vi "TCP Client_34.vi"(0 "CMD":i32(ring) items=["OCP_IF_CMD_TRACE_READ", "OCP_IF_CMD_TRACE_RESET", "OCP_IF_CMD_TRACE_GET_SIZE", "OCP_IF_CMD_TRACE_SET_SIZE", "OCP_IF_CMD_TRACE_GET_NUMBER_SIGNALS", "OCP_IF_CMD_TRACE_GET_SIGNALS_NAMES", "OCP_IF_CMD_TRACE_GET_NUMBER_TRACES", "OCP_IF_CMD_TRACE_GET_TRACES_NAMES", "OCP_IF_CMD_TRACE_GET_ADDRESS", "OCP_IF_CMD_CS_STATUS", "OCP_IF_CMD_CS_ENABLE", "OCP_IF_CMD_CS_DISABLE", "OCP_IF_CMD_CS_CONTROLLER_IF", "OCP_IF_CMD_CS_HARDWARE_IF", "OCP_IF_CMD_CS_GET_NUMBER_CONTROLLERS", "OCP_IF_CMD_CS_GET_CONTROLLERS_NAMES", "OCP_IF_CMD_PLATFORM_ID", "OCP_IF_CMD_PLATFORM_IF", "OCP_IF_CMD_OPIL_UPDATE_MEASUREMENTS", "OCP_IF_CMD_OPIL_UPDATE_SIM_DATA", "OCP_IF_CMD_OPIL_RUN_CONTROL", "OCP_IF_CMD_OPIL_INITIALIZE_CONTROL", "OCP_IF_CMD_OPIL_GET_CONTROL", "OCP_IF_CMD_OPIL_GET_CONTROLLER_DATA", "OCP_IF_CMD_END"], 2 "Input Cluster":T3, 3 "error in (no error)":errorcluster, 8 "Comunication Cluster":T1) -> (6 "Output cluster":T2, 7 "R_message 1":string, 10 "error out":errorcluster)   [LabVIEW 2021]
uses:
  <vilib>/ErrorRing/Error Ring.xnode
  <vilib>/Utility/error.llb/Error Cluster From Error Code.vi
panel:
  out "R_Data string length":cluster{i32}
  out "W_Data string length: \nbytes written 2":i32
  out "W_Data string_flat":string
  # "0-> OCP_IF_CMD_TRACE_READ = 0, //LV: SIZE - CMD - ID || RESPONSE: SIZE - DATA\n1->\tOCP_IF_CMD_TRACE_RESET, //SIZE - CMD - ID || RESPONSE: SIZE\n2-> OCP_IF_CMD_TRACE_GET_SIZE, //SIZE - CMD - ID || RESPONSE: SIZE - TRACE_SIZE (4 bztes)\n3->\tOCP_IF_CMD_TRACE_SET_SIZE, //SIZE - CMD - ID - TRACE_SIZE ( 4 bytes) || RESPONSE: SIZE\n4->\tOCP_IF_CMD_TRACE_GET_NUMBER_SIGNALS, //SIZE - CMD - ID || RESPONSE: SIZE - NB_SIGNALS (4 bytes)\n5->\tOCP_IF_CMD_TRACE_GET_SIGNALS_NAMES, //SIZE - CMD - ID || RESPONSE: SIZE - string\n6->\tOCP_IF_CMD_TRACE_GET_NUMBER_TRACES, //SIZE - CMD  || RESPONSE: SIZE - NB_TRACES (4 bytes)\n7->\tOCP_IF_CMD_TRACE_GET_TRACES_NAMES, //SIZE - CMD || RESPONSE: SIZE - NB_TRACES (N bytes)\n8-> OCP_IF_CMD_TRACE_GET_ADDRESS, //SIZE - CMD - ID || RESPONSE: SIZE - TRACE ADDRESS (4 bytes)\n9-> OCP_IF_CMD_CS_STATUS, //SIZE - CMD - ID || RESPONSE: SIZE - CS STATUS (4 bytes)\n10-> OCP_IF_CMD_CS_ENABLE, //SIZE - CMD - ID || RESPONSE: SIZE\n11-> OCP_IF_CMD_CS_DISABLE, //SIZE - CMD - ID || RESPONSE: SIZE\n12-> OCP_IF_CMD_CS_CONTROLLER_IF, //SIZE - CMD - ID - DATA (N) || RESPONSE: SIZE - DATA (M)\n13-> OCP_IF_CMD_CS_HARDWARE_IF, //SIZE - CMD - ID - DATA (N) || RESPONSE: SIZE - DATA (M)\n14-> OCP_IF_CMD_CS_GET_NUMBER_CONTROLLERS, //SIZE - CMD || RESPONSE: SIZE - NB CSs\n15-> OCP_IF_CMD_CS_GET_CONTROLLERS_NAMES, //SIZE - CMD || RESPONSE: SIZE - string NAMES CSs"
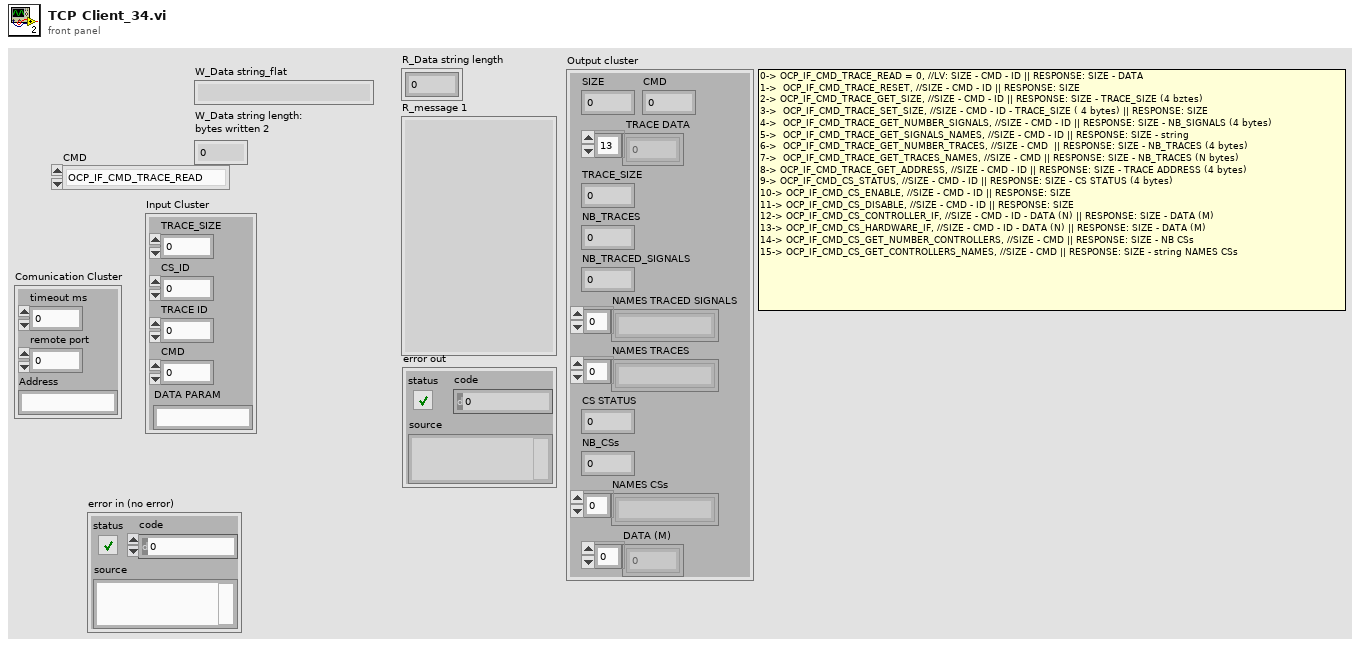
[diagram p1: front panel]
types:
  T1 = cluster{"timeout ms":i32, "remote port":u16, "Address":string}
  T2 = cluster{"SIZE":i32, " TRACE DATA":sgl[], "TRACE_SIZE":i32, "NB_TRACES":i32, "NB_TRACED_SIGNALS":i32, "NAMES TRACED SIGNALS":string[], "NAMES TRACES":string[], "CS STATUS":i32, "NB_CSs":i32, "NAMES CSs":string[], "DATA (M)":sgl[], "CMD":i32}
  T3 = cluster{"TRACE_SIZE":i32, "CS_ID":i32, "TRACE ID":i32, "CMD":i32, "DATA PARAM":string}
  T4 = enum16{"big-endian, network order", "native, host order", "little-endian"}
  T5 = enum16{"Standard", "Buffered", "CRLF", "Immediate"}
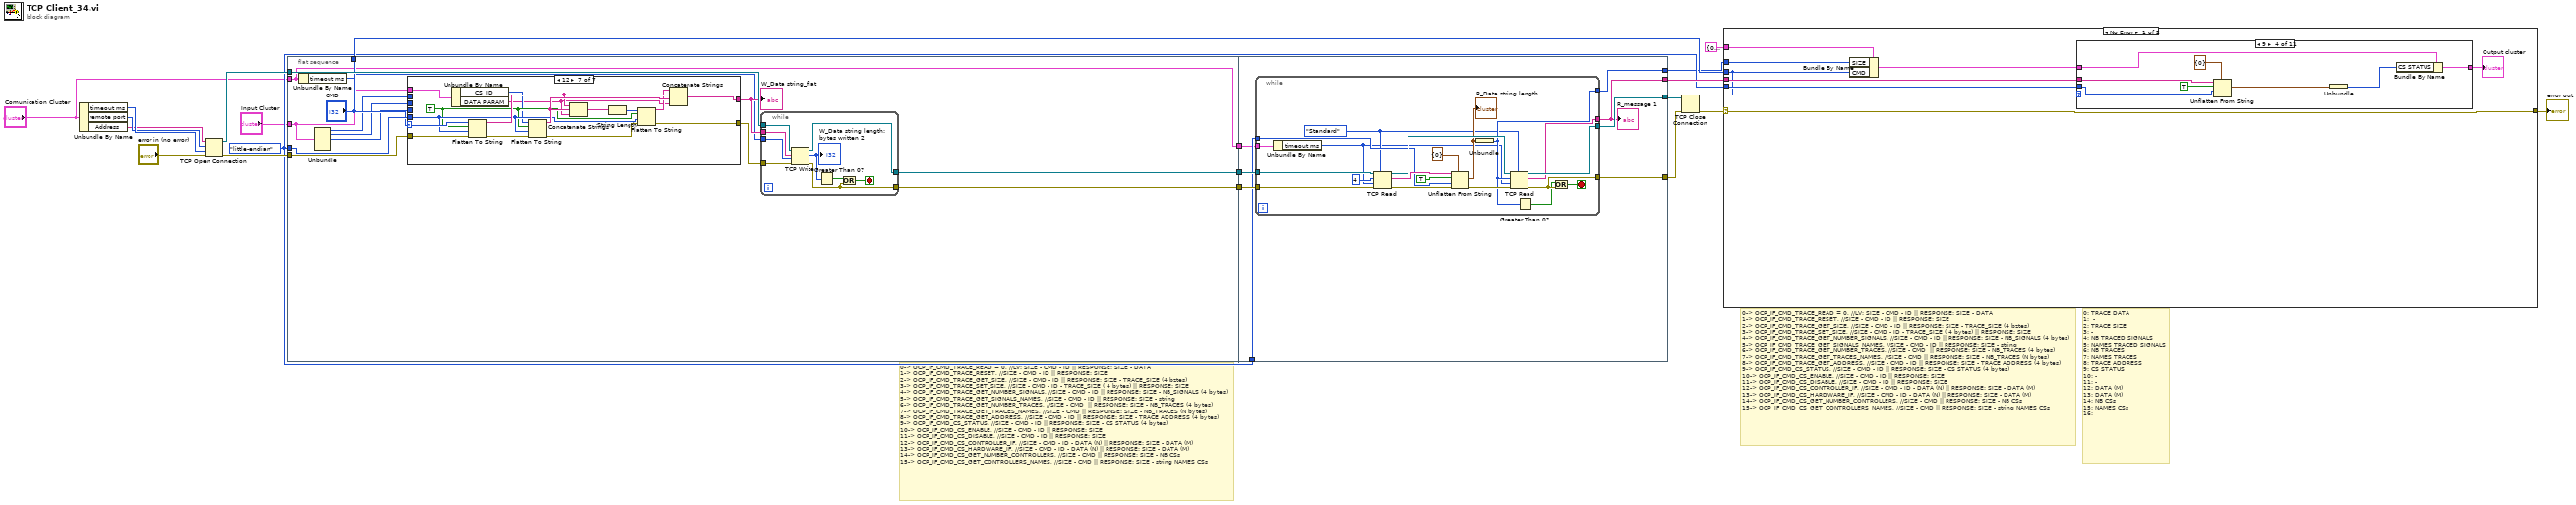
[diagram p0: block diagram]
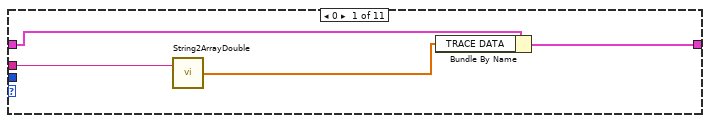
[diagram p2: hidden frame]
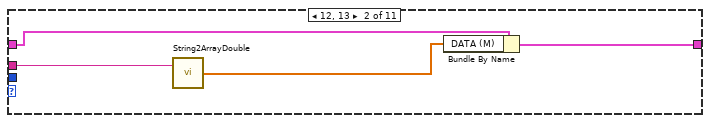
[diagram p3: hidden frame]
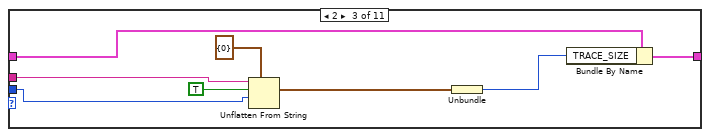
[diagram p4: hidden frame]
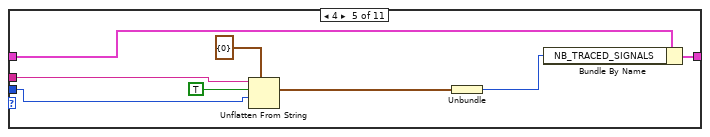
[diagram p5: hidden frame]
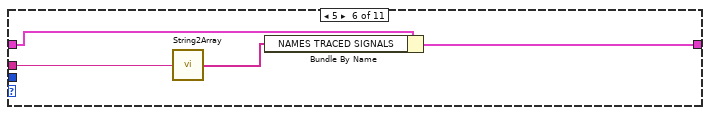
[diagram p6: hidden frame]
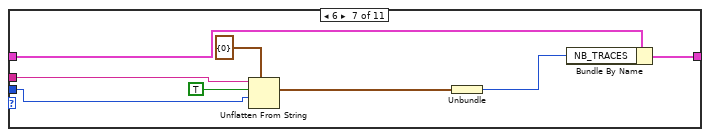
[diagram p7: hidden frame]
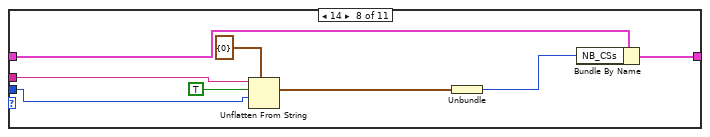
[diagram p8: hidden frame]
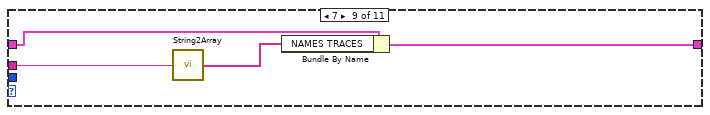
[diagram p9: hidden frame]
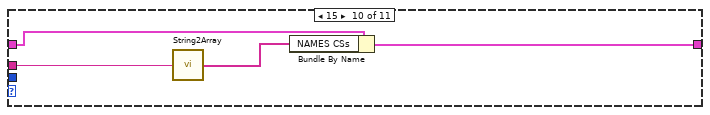
[diagram p10: hidden frame]
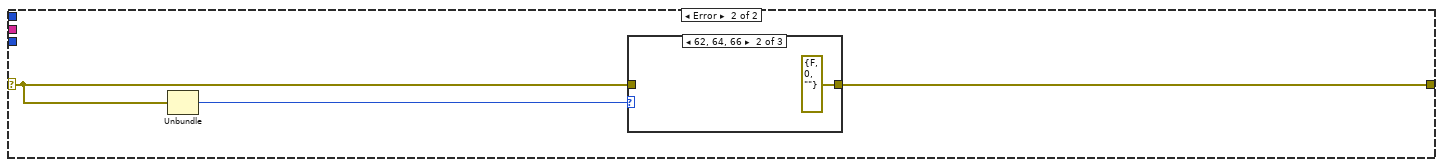
[diagram p12: hidden frame]
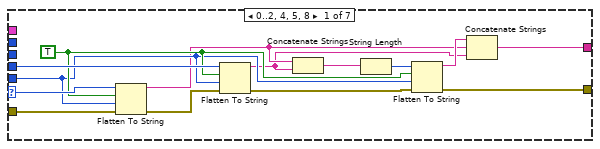
[diagram p15: hidden frame]
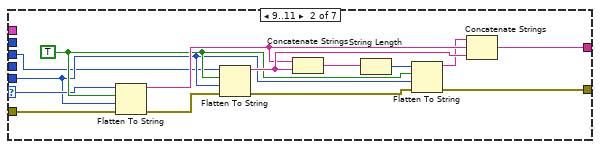
[diagram p16: hidden frame]
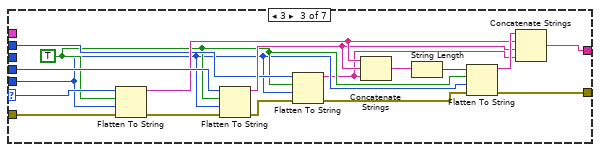
[diagram p17: hidden frame]
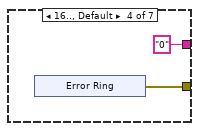
[diagram p18: hidden frame]
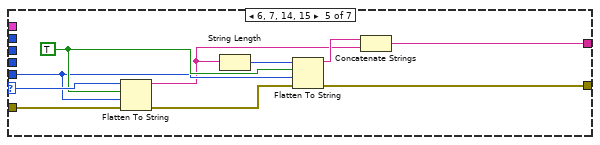
[diagram p19: hidden frame]
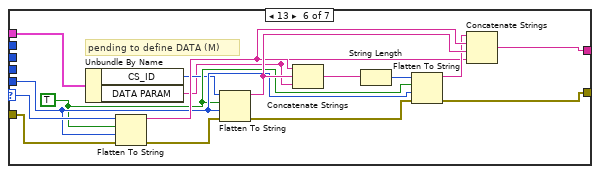
[diagram p20: hidden frame]
diagram:
  w8 = T4."little-endian" ("byte order (0:big-endian, network order)")
  # "0-> OCP_IF_CMD_TRACE_READ = 0, //LV: SIZE - CMD - ID || RESPONSE: SIZE - DATA\n1->\tOCP_IF_CMD_TRACE_RESET, //SIZE - CMD - ID || RESPONSE: SIZE\n2-> OCP_IF_CMD_TRACE_GET_SIZE, //SIZE - CMD - ID || RESPONSE: SIZE - TRACE_SIZE (4 bztes)\n3->\tOCP_IF_CMD_TRACE_SET_SIZE, //SIZE - CMD - ID - TRACE_SIZE ( 4 bytes) || RESPONSE: SIZE\n4->\tOCP_IF_CMD_TRACE_GET_NUMBER_SIGNALS, //SIZE - CMD - ID || RESPONSE: SIZE - NB_SIGNALS (4 bytes)\n5->\tOCP_IF_CMD_TRACE_GET_SIGNALS_NAMES, //SIZE - CMD - ID || RESPONSE: SIZE - string\n6->\tOCP_IF_CMD_TRACE_GET_NUMBER_TRACES, //SIZE - CMD  || RESPONSE: SIZE - NB_TRACES (4 bytes)\n7->\tOCP_IF_CMD_TRACE_GET_TRACES_NAMES, //SIZE - CMD || RESPONSE: SIZE - NB_TRACES (N bytes)\n8-> OCP_IF_CMD_TRACE_GET_ADDRESS, //SIZE - CMD - ID || RESPONSE: SIZE - TRACE ADDRESS (4 bytes)\n9-> OCP_IF_CMD_CS_STATUS, //SIZE - CMD - ID || RESPONSE: SIZE - CS STATUS (4 bytes)\n10-> OCP_IF_CMD_CS_ENABLE, //SIZE - CMD - ID || RESPONSE: SIZE\n11-> OCP_IF_CMD_CS_DISABLE, //SIZE - CMD - ID || RESPONSE: SIZE\n12-> OCP_IF_CMD_CS_CONTROLLER_IF, //SIZE - CMD - ID - DATA (N) || RESPONSE: SIZE - DATA (M)\n13-> OCP_IF_CMD_CS_HARDWARE_IF, //SIZE - CMD - ID - DATA (N) || RESPONSE: SIZE - DATA (M)\n14-> OCP_IF_CMD_CS_GET_NUMBER_CONTROLLERS, //SIZE - CMD || RESPONSE: SIZE - NB CSs\n15-> OCP_IF_CMD_CS_GET_CONTROLLERS_NAMES, //SIZE - CMD || RESPONSE: SIZE - string NAMES CSs"
  # "0: TRACE DATA\n1:  -\n2: TRACE SIZE\n3: -\n4: NB TRACED SIGNALS\n5: NAMES TRACED SIGNALS\n6: NB TRACES\n7: NAMES TRACES\n8: TRACE ADDRESS\n9: CS STATUS\n10: -\n11: -\n12: DATA (M)\n13: DATA (M)\n14: NB CSs \n15: NAMES CSs \n16:"
  # "0-> OCP_IF_CMD_TRACE_READ = 0, //LV: SIZE - CMD - ID || RESPONSE: SIZE - DATA\n1->\tOCP_IF_CMD_TRACE_RESET, //SIZE - CMD - ID || RESPONSE: SIZE\n2-> OCP_IF_CMD_TRACE_GET_SIZE, //SIZE - CMD - ID || RESPONSE: SIZE - TRACE_SIZE (4 bztes)\n3->\tOCP_IF_CMD_TRACE_SET_SIZE, //SIZE - CMD - ID - TRACE_SIZE ( 4 bytes) || RESPONSE: SIZE\n4->\tOCP_IF_CMD_TRACE_GET_NUMBER_SIGNALS, //SIZE - CMD - ID || RESPONSE: SIZE - NB_SIGNALS (4 bytes)\n5->\tOCP_IF_CMD_TRACE_GET_SIGNALS_NAMES, //SIZE - CMD - ID || RESPONSE: SIZE - string\n6->\tOCP_IF_CMD_TRACE_GET_NUMBER_TRACES, //SIZE - CMD  || RESPONSE: SIZE - NB_TRACES (4 bytes)\n7->\tOCP_IF_CMD_TRACE_GET_TRACES_NAMES, //SIZE - CMD || RESPONSE: SIZE - NB_TRACES (N bytes)\n8-> OCP_IF_CMD_TRACE_GET_ADDRESS, //SIZE - CMD - ID || RESPONSE: SIZE - TRACE ADDRESS (4 bytes)\n9-> OCP_IF_CMD_CS_STATUS, //SIZE - CMD - ID || RESPONSE: SIZE - CS STATUS (4 bytes)\n10-> OCP_IF_CMD_CS_ENABLE, //SIZE - CMD - ID || RESPONSE: SIZE\n11-> OCP_IF_CMD_CS_DISABLE, //SIZE - CMD - ID || RESPONSE: SIZE\n12-> OCP_IF_CMD_CS_CONTROLLER_IF, //SIZE - CMD - ID - DATA (N) || RESPONSE: SIZE - DATA (M)\n13-> OCP_IF_CMD_CS_HARDWARE_IF, //SIZE - CMD - ID - DATA (N) || RESPONSE: SIZE - DATA (M)\n14-> OCP_IF_CMD_CS_GET_NUMBER_CONTROLLERS, //SIZE - CMD || RESPONSE: SIZE - NB CSs\n15-> OCP_IF_CMD_CS_GET_CONTROLLERS_NAMES, //SIZE - CMD || RESPONSE: SIZE - string NAMES CSs"
  n1 = Unbundle By Name("Comunication Cluster") -> ("timeout ms"=w4:i32, "remote port"=w3:u16, "Address"=w2:string)
  n2 = TCP Open Connection(address=w2, remote port or service name=w3, timeout ms (60000)=w4, error in (no error)="error in (no error)") -> (connection ID=w20:refnum<k5>, error out=w19:errorcluster)  [unwired: 1 in]
  n3 = flat-sequence {
    tunnel: w20 -> [w34]
    tunnel: w19 -> [w31]
    tunnel: [w33] -> w18
    tunnel: [w32] -> w17
    tunnel: w8 -> [w30]
    tunnel: ["CMD"] -> w11
    tunnel: "Input Cluster" -> [w24]
    tunnel: "Comunication Cluster" -> [w22]
    tunnel: [w22] -> w1
    tunnel: w18 -> [w145]
    tunnel: w17 -> [w144]
    tunnel: [w143] -> w14
    tunnel: [w142] -> w13
    tunnel: w8 -> [w141]
    tunnel: [w140] -> w10
    tunnel: [w139] -> w7
    tunnel: w1 -> [w138]
    frame #0 {
      n4 = Unbundle By Name(w22) -> ("timeout ms"=w23:i32)
      n5 = Unbundle(w24) -> ("TRACE_SIZE"=w25:i32, "CS_ID"=w27:i32, "TRACE ID"=w26:i32)  [unwired: 2 out]
      n6 = case shown="12" "CMD" {
        selector: "CMD" -> [w55 w62 w86 _ w104 w113 w129]
        tunnel: w31 -> [w57 w63 w88 _ w105 w112 w128]
        tunnel: w30 -> [w48 w61 w74 _ w100 w109 w125]
        tunnel: w26 -> [w54 _ w85 _ _ _ _]
        tunnel: [w47 w59 w81 "0" w99 w115 w131] -> w29
        tunnel: [w46 w58 w73 w90 w97 w114 w130] -> w21
        tunnel: w25 -> [_ _ w76 _ _ _ _]
        tunnel: w27 -> [_ w60 _ _ _ _ _]
        tunnel: w24 -> [_ _ _ _ _ w111 w127]
        frame 0..2, 4, 5, 8 {
          w49 = TRUE ("prepend array or string size? (T)")
          n7 = Flatten To String(anything=w55, prepend array or string size? (T)=w49, byte order (0:big-endian, network order)=w48, error in (no error)=w57) -> (data string=w45:string, error out=w56:errorcluster)  [unwired: 1 out]
          n8 = Flatten To String(anything=w54, prepend array or string size? (T)=w49, byte order (0:big-endian, network order)=w48, error in (no error)=w56) -> (data string=w44:string, error out=w51:errorcluster)  [unwired: 1 out]
          n9 = Concatenate Strings(w45, w44) -> (w53:string)
          n10 = String Length(string=w53) -> (length=w52:i32)
          n11 = Flatten To String(anything=w52, prepend array or string size? (T)=w49, byte order (0:big-endian, network order)=w48, error in (no error)=w51) -> (data string=w50:string, error out=w46:errorcluster)  [unwired: 1 out]
          n12 = Concatenate Strings(w50, w45, w44) -> (w47:string)
        }
        frame 9..11 {
          w64 = TRUE ("prepend array or string size? (T)")
          n13 = Flatten To String(anything=w62, prepend array or string size? (T)=w64, byte order (0:big-endian, network order)=w61, error in (no error)=w63) -> (data string=w70:string, error out=w65:errorcluster)  [unwired: 1 out]
          n14 = Flatten To String(anything=w60, prepend array or string size? (T)=w64, byte order (0:big-endian, network order)=w61, error in (no error)=w65) -> (data string=w71:string, error out=w68:errorcluster)  [unwired: 1 out]
          n15 = Concatenate Strings(w70, w71) -> (w66:string)
          n16 = String Length(string=w66) -> (length=w67:i32)
          n17 = Flatten To String(anything=w67, prepend array or string size? (T)=w64, byte order (0:big-endian, network order)=w61, error in (no error)=w68) -> (data string=w69:string, error out=w58:errorcluster)  [unwired: 1 out]
          n18 = Concatenate Strings(w69, w70, w71) -> (w59:string)
        }
        frame 3 {
          w75 = TRUE ("prepend array or string size? (T)")
          n19 = Flatten To String(anything=w86, prepend array or string size? (T)=w75, byte order (0:big-endian, network order)=w74, error in (no error)=w88) -> (data string=w80:string, error out=w87:errorcluster)  [unwired: 1 out]
          n20 = Flatten To String(anything=w85, prepend array or string size? (T)=w75, byte order (0:big-endian, network order)=w74, error in (no error)=w87) -> (data string=w79:string, error out=w78:errorcluster)  [unwired: 1 out]
          n21 = Flatten To String(anything=w76, prepend array or string size? (T)=w75, byte order (0:big-endian, network order)=w74, error in (no error)=w78) -> (data string=w72:string, error out=w77:errorcluster)  [unwired: 1 out]
          n22 = Concatenate Strings(w80, w79, w72) -> (w84:string)
          n23 = String Length(string=w84) -> (length=w83:i32)
          n24 = Flatten To String(anything=w83, prepend array or string size? (T)=w75, byte order (0:big-endian, network order)=w74, error in (no error)=w77) -> (data string=w82:string, error out=w73:errorcluster)  [unwired: 1 out]
          n25 = Concatenate Strings(w82, w80, w79, w72) -> (w81:string)
        }
        frame 16.., Default {
          n26 = xnode "Error Ring"() -> ("error out"=w90:errorcluster)
        }
        frame 6, 7, 14, 15 {
          w101 = TRUE ("prepend array or string size? (T)")
          n27 = Flatten To String(anything=w104, prepend array or string size? (T)=w101, byte order (0:big-endian, network order)=w100, error in (no error)=w105) -> (data string=w96:string, error out=w98:errorcluster)  [unwired: 1 out]
          n28 = String Length(string=w96) -> (length=w103:i32)
          n29 = Flatten To String(anything=w103, prepend array or string size? (T)=w101, byte order (0:big-endian, network order)=w100, error in (no error)=w98) -> (data string=w102:string, error out=w97:errorcluster)  [unwired: 1 out]
          n30 = Concatenate Strings(w102, w96) -> (w99:string)
        }
        frame 13 {
          w108 = TRUE ("prepend array or string size? (T)")
          # "pending to define DATA (M)"
          n31 = Unbundle By Name(w111) -> ("CS_ID"=w107:i32, "DATA PARAM"=w106:string)
          n32 = Flatten To String(anything=w113, prepend array or string size? (T)=w108, byte order (0:big-endian, network order)=w109, error in (no error)=w112) -> (data string=w120:string, error out=w116:errorcluster)  [unwired: 1 out]
          n33 = Flatten To String(anything=w107, prepend array or string size? (T)=w108, byte order (0:big-endian, network order)=w109, error in (no error)=w116) -> (data string=w121:string, error out=w110:errorcluster)  [unwired: 1 out]
          n34 = Concatenate Strings(w120, w121, w106) -> (w117:string)
          n35 = String Length(string=w117) -> (length=w118:i32)
          n36 = Flatten To String(anything=w118, prepend array or string size? (T)=w108, byte order (0:big-endian, network order)=w109, error in (no error)=w110) -> (data string=w119:string, error out=w114:errorcluster)  [unwired: 1 out]
          n37 = Concatenate Strings(w119, w120, w121, w106) -> (w115:string)
        }
        frame 12 {
          w124 = TRUE ("prepend array or string size? (T)")
          n38 = Unbundle By Name(w127) -> ("CS_ID"=w123:i32, "DATA PARAM"=w122:string)
          n39 = Flatten To String(anything=w129, prepend array or string size? (T)=w124, byte order (0:big-endian, network order)=w125, error in (no error)=w128) -> (data string=w136:string, error out=w132:errorcluster)  [unwired: 1 out]
          n40 = Flatten To String(anything=w123, prepend array or string size? (T)=w124, byte order (0:big-endian, network order)=w125, error in (no error)=w132) -> (data string=w137:string, error out=w126:errorcluster)  [unwired: 1 out]
          n41 = Concatenate Strings(w136, w137, w122) -> (w133:string)
          n42 = String Length(string=w133) -> (length=w134:i32)
          n43 = Flatten To String(anything=w134, prepend array or string size? (T)=w124, byte order (0:big-endian, network order)=w125, error in (no error)=w126) -> (data string=w135:string, error out=w130:errorcluster)  [unwired: 1 out]
          n44 = Concatenate Strings(w135, w136, w137, w122) -> (w131:string)
        }
      }
      "W_Data string_flat" <- w29
      n45 = while {
        tunnel: w29 -> [w41]
        tunnel: w23 -> [w40]
        tunnel: w21 -> [w39]
        tunnel: [w37] -> w33
        tunnel: w34 -> [w43]
        tunnel: [w42] -> w32
        stop <- w38 stop-if-true
        n46 = TCP Write(connection ID=w43, data in=w41, error in (no error)=w39, 9:w40) -> (connection ID out=w42:refnum<k5>, bytes written=w36:i32, error out=w37:errorcluster)
        "W_Data string length: \nbytes written 2" <- w36
        n47 = Greater Than 0?(x=w36) -> (x > 0?=w35:bool)
        n48 = Or(x=w35, y=w37) -> (x .or. y?=w38:bool)
      }
    }
    frame #1 {
      n49 = while {
        tunnel: w141 -> [w155]
        tunnel: [w153] -> w140
        tunnel: [w150] -> w139
        tunnel: w144 -> [w163]
        tunnel: [w162] -> w143
        tunnel: w145 -> [w164]
        tunnel: [w152] -> w142
        tunnel: w138 -> [w146]
        stop <- w151 stop-if-true
        w148 = T5."Standard" ("mode (standard)")
        n50 = Unbundle By Name(w146) -> ("timeout ms"=w147:i32)
        n51 = TCP Read(connection ID=w163, bytes to read=4, error in (no error)=w164, 7:w148, 9:w147) -> (connection ID out=w165:refnum<k5>, data out=w161:string, error out=w157:errorcluster)
        n52 = Unflatten From String(type=cluster{i32} {0}, binary string=w161, data includes array or string size? (T)=TRUE, byte order (0:big-endian, network order)=w155, error in (no error)=w157) -> (value=w158:cluster{i32}, error out=w156:errorcluster)  [unwired: 1 out]
        "R_Data string length" <- w158
        n53 = Unbundle(w158) -> (w150:i32)
        n54 = TCP Read(connection ID=w165, bytes to read=w150, error in (no error)=w156, 7:w148, 9:w147) -> (connection ID out=w162:refnum<k5>, data out=w153:string, error out=w152:errorcluster)
        n55 = Greater Than 0?(x=w150) -> (x > 0?=w149:bool)
        n56 = Or(x=w149, y=w152) -> (x .or. y?=w151:bool)
      }
      "R_message 1" <- w140
    }
  }
  n57 = TCP Close Connection(connection ID=w14, error in (no error)=w13) -> (error out=w15:errorcluster)  [unwired: 1 in, 1 out]
  n58 = case shown="No Error" w15 {
    selector: w15 -> [w173 w236]
    tunnel: [w173 w235] -> w16
    tunnel: w11 -> [w167 _]
    tunnel: w10 -> [w169 _]
    tunnel: T2 {"SIZE"=0, " TRACE DATA"=[], "TRACE_SIZE"=0, "NB_TRACES"=0, "NB_TRACED_SIGNALS"=0, "NAMES TRACED SIGNALS"=[], "NAMES TRACES"=[], "CS STATUS"=0, "NB_CSs"=0, "NAMES CSs"=[], "DATA (M)"=[], "CMD"=0} ("input cluster") -> [w172 _]
    tunnel: w8 -> [w168 _]
    tunnel: w7 -> [w170 _]
    frame No Error {
      n59 = Bundle By Name(cluster=w172, "SIZE"=w170, "CMD"=w167) -> (w171:T2)
      n60 = case shown="9" w167 {
        tunnel: [w176 w180 w188 w196 w204 w208 w217 w225 w228 w232 w234] -> w166
        tunnel: w171 -> [w177 w181 w189 w197 w205 w209 w214 w222 w229 w233 w234]
        tunnel: w169 -> [w174 w178 w186 w194 w201 w207 w212 w220 w227 w231 _]
        tunnel: w168 -> [_ _ w184 w192 w200 _ w213 w221 _ _ _]
        frame 0 {
          n61 = call "String2ArrayDouble.vi"("R_message 1"=w174) -> ("Array"=w175:sgl[])  [unwired: 1 in]
          n62 = Bundle By Name(cluster=w177, "TRACE DATA"=w175) -> (w176:T2)
        }
        frame 12, 13 {
          n63 = call "String2ArrayDouble.vi"("R_message 1"=w178) -> ("Array"=w179:sgl[])  [unwired: 1 in]
          n64 = Bundle By Name(cluster=w181, "DATA (M)"=w179) -> (w180:T2)
        }
        frame 2 {
          n65 = Unflatten From String(type=cluster{i32} {0}, binary string=w186, data includes array or string size? (T)=TRUE, byte order (0:big-endian, network order)=w184) -> (value=w183:cluster{i32})  [unwired: 1 in, 2 out]
          n66 = Unbundle(w183) -> (w182:i32)
          n67 = Bundle By Name(cluster=w189, "TRACE_SIZE"=w182) -> (w188:T2)
        }
        frame 9 {
          n68 = Unflatten From String(type=cluster{i32} {0}, binary string=w194, data includes array or string size? (T)=TRUE, byte order (0:big-endian, network order)=w192) -> (value=w191:cluster{i32})  [unwired: 1 in, 2 out]
          n69 = Unbundle(w191) -> (w190:i32)
          n70 = Bundle By Name(cluster=w197, "CS STATUS"=w190) -> (w196:T2)
        }
        frame 4 {
          n71 = Unflatten From String(type=cluster{i32} {0}, binary string=w201, data includes array or string size? (T)=TRUE, byte order (0:big-endian, network order)=w200) -> (value=w202:cluster{i32})  [unwired: 1 in, 2 out]
          n72 = Unbundle(w202) -> (w198:i32)
          n73 = Bundle By Name(cluster=w205, "NB_TRACED_SIGNALS"=w198) -> (w204:T2)
        }
        frame 5 {
          n74 = call "String2Array.vi"("R_message 1"=w207) -> ("Array 2"=w206:string[])
          n75 = Bundle By Name(cluster=w209, "NAMES TRACED SIGNALS"=w206) -> (w208:T2)
        }
        frame 6 {
          n76 = Unflatten From String(type=cluster{i32} {0}, binary string=w212, data includes array or string size? (T)=TRUE, byte order (0:big-endian, network order)=w213) -> (value=w216:cluster{i32})  [unwired: 1 in, 2 out]
          n77 = Unbundle(w216) -> (w210:i32)
          n78 = Bundle By Name(cluster=w214, "NB_TRACES"=w210) -> (w217:T2)
        }
        frame 14 {
          n79 = Unflatten From String(type=cluster{i32} {0}, binary string=w220, data includes array or string size? (T)=TRUE, byte order (0:big-endian, network order)=w221) -> (value=w224:cluster{i32})  [unwired: 1 in, 2 out]
          n80 = Unbundle(w224) -> (w218:i32)
          n81 = Bundle By Name(cluster=w222, "NB_CSs"=w218) -> (w225:T2)
        }
        frame 7 {
          n82 = call "String2Array.vi"("R_message 1"=w227) -> ("Array 2"=w226:string[])
          n83 = Bundle By Name(cluster=w229, "NAMES TRACES"=w226) -> (w228:T2)
        }
        frame 15 {
          n84 = call "String2Array.vi"("R_message 1"=w231) -> ("Array 2"=w230:string[])
          n85 = Bundle By Name(cluster=w233, "NAMES CSs"=w230) -> (w232:T2)
        }
        frame 8, Default {
        }
      }
      "Output cluster" <- w166
    }
    frame Error {
      n86 = Unbundle(w236) -> ("code"=w237:i32)  [unwired: 2 out]
      n87 = case shown="62, 64, 66" w237 {
        tunnel: [w238 errorcluster {"status"=FALSE, "code"=0, "source"=""} ("error IO") w240] -> w235
        tunnel: w236 -> [w238 _ w240]
        frame 0, Default {
        }
        frame 62, 64, 66 {
        }
        frame 56 {
        }
      }
    }
  }
  "error out" <- w16
